vi "Poly_ReadDigitalIn.vi"   [LabVIEW 2012]
doc: "Reads the specified digitial \"Channel\" and returns the retrieved value as \"Variable Out\"."
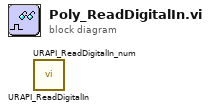
[diagram p0: block diagram]
diagram:
  n1 = call <userlib>:"URAPI_ReadDigitalIn.vi"() -> ()  [unwired: 4 in, 2 out]
  n2 = call <userlib>:"URAPI_ReadDigitalIn_num.vi"() -> ()  [unwired: 4 in, 2 out]
